vi "Read Ai Average.vi"(0 "FPGA API in":refnum<class "FPGA API.lvclass">, 11 "error in (no error)":errorcluster) -> (4 "FPGA API out":refnum<class "FPGA API.lvclass">, 6 "Raw":T1, 8 "Average 1ms":T1, 10 "Discrete Control Filter":T1, 15 "error out":errorcluster)   [LabVIEW 2019, in "FPGA API.lvclass"]
uses:
  FPGA API.lvclass
  FPGA API.lvclass/FPGA API.ctl
  <vilib>/Utility/error.llb/Error Cluster From Error Code.vi
  <vilib>/rvi/errors/niLvFpgaAdjustHostInterfaceError.vi
  <vilib>/rvi/interface/nirviReadWriteControl/nirviReadWriteControl.xnode
  FPGA Ref.ctl
  NiFpgaLv.dll
  <vilib>/rvi/interface/Simulation/niFpgaSimulationCallBeginRW.vi
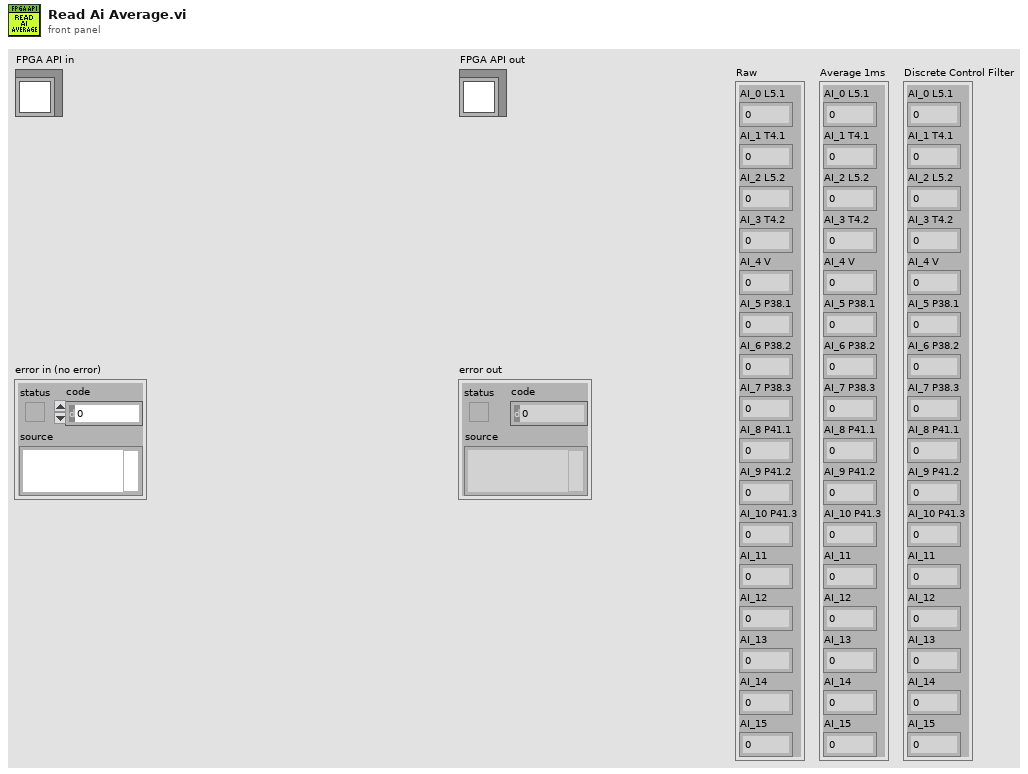
[diagram p1: front panel]
types:
  T1 = cluster{"AI_0 L5.1":fxp<+/-,21,-4>, "AI_1 T4.1":fxp<+/-,21,-4>, "AI_2 L5.2":fxp<+/-,21,-4>, "AI_3 T4.2":fxp<+/-,21,-4>, "AI_4 V":fxp<+/-,21,-4>, "AI_5 P38.1":fxp<+/-,21,-4>, "AI_6 P38.2":fxp<+/-,21,-4>, "AI_7 P38.3":fxp<+/-,21,-4>, "AI_8 P41.1":fxp<+/-,21,-4>, "AI_9 P41.2":fxp<+/-,21,-4>, "AI_10 P41.3":fxp<+/-,21,-4>, "AI_11":fxp<+/-,21,-4>, "AI_12":fxp<+/-,21,-4>, "AI_13":fxp<+/-,21,-4>, "AI_14":fxp<+/-,21,-4>, "AI_15":fxp<+/-,21,-4>}
  T2 = typedef "FPGA API.lvclass/FPGA Ref.ctl" = refnum<k20>
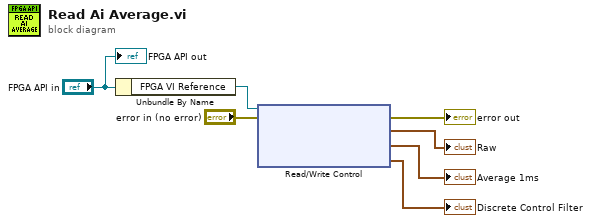
[diagram p0: block diagram]
diagram:
  n1 = Unbundle By Name("FPGA API in") -> ("FPGA VI Reference"=w6:T2)
  n2 = xnode "Read/Write Control"("FPGA VI Reference In"=w6, "error in"="error in (no error)") -> ("error out"=→"error out":errorcluster, "Raw"=→"Raw":T1, "Average 1ms"=→"Average 1ms":T1, "Discrete Control Filter"=→"Discrete Control Filter":T1)  [unwired: 1 out]
  "FPGA API out" <- "FPGA API in"
